vi "User-Defined IO Variable - Basic.vi"   [LabVIEW 2015]
uses:
  <vilib>/rvi/Emulation/niFpgaGetClockAttributes.vi
  <vilib>/rvi/Emulation/niFpgaSctlEmulationGetInTimedLoop.vi
  <vilib>/rvi/Emulation/niFpgaEmulationReportErrorSimple.vi
  <vilib>/rvi/Emulation/niFpgaCriticalErrorInLSC.vi
panel:
  # "See block diagram"
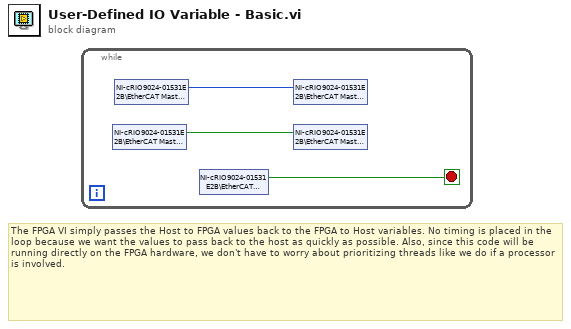
[diagram p0: block diagram]
diagram:
  # "The FPGA VI simply passes the Host to FPGA values back to the FPGA to Host variables. No timing is placed in the loop because we want the values to pass back to the host as quickly as possible. Also, since this code will be running directly on the FPGA hardware, we don't have to worry about prioritizing threads like we do if a processor is involved."
  n1 = while {
    stop <- w1 stop-if-true
    n2 = shared-variable "NI-cRIO9024-01531E2B\\EtherCAT Master\\Device\\User-Defined Variables\\HFBo"() -> (w3:bool)  [unwired: 1 in, 1 out]
    n3 = shared-variable "NI-cRIO9024-01531E2B\\EtherCAT Master\\Device\\User-Defined Variables\\HFInt"() -> (w2:i32)  [unwired: 1 in, 1 out]
    n4 = shared-variable "NI-cRIO9024-01531E2B\\EtherCAT Master\\Device\\User-Defined Variables\\Stop"() -> (w1:bool)  [unwired: 1 in, 1 out]
    n5 = shared-variable "NI-cRIO9024-01531E2B\\EtherCAT Master\\Device\\User-Defined Variables\\FHInt"(w2) -> ()  [unwired: 1 in, 1 out]
    n6 = shared-variable "NI-cRIO9024-01531E2B\\EtherCAT Master\\Device\\User-Defined Variables\\FHBo"(w3) -> ()  [unwired: 1 in, 1 out]
  }
